vi "5492_WPI_RobotDriveArcadeDrive_Standard(NoSaturation).vi"(0 "RobotDriveDevRef":T1={"DevStatus"={"status"=FALSE, "code"=0, "source"=""}, "Motors[]"=[], "Square Inputs"=FALSE, "Max Output"=1.0}, 5 "X axis value":dbl, 7 "Orientation Toggle":bool, 9 "Y axis value":dbl, 11 "error in (no error)":errorcluster) -> (4 "RobotDriveDevRef":T1={"DevStatus"={"status"=FALSE, "code"=0, "source"=""}, "Motors[]"=[], "Square Inputs"=FALSE, "Max Output"=1.0}, 6 "Motor Values":dbl[](array[numeric]), 15 "error out":errorcluster)   [LabVIEW 2016]
doc: "Uses a standard algorithm to configure the motors for arcade driving. This algorithm does not saturate over half of the range.\n\nThis software is licensed. Open the labview\\readme\\WPI Robotics Library Open Source License.txt file for more information."
uses:
  <vilib>/Rock Robotics/WPI/RobotDrive/WPI_RobotDriveDevRef.ctl
  <vilib>/Rock Robotics/WPI/MotorControl/WPI_MotorControlDeviceRef.ctl
  <vilib>/Rock Robotics/WPI/MotorControl/WPI_MotorControlType.ctl
  <vilib>/Rock Robotics/SystemInterfaces/DIO/FPGA_DIOPWMChannel.ctl
  <vilib>/Rock Robotics/WPI/PWM/WPI_PWMDeadband.ctl
  <vilib>/Rock Robotics/SystemInterfaces/NetworkCommunication/NetComm_UsageReport_ResourceType.ctl
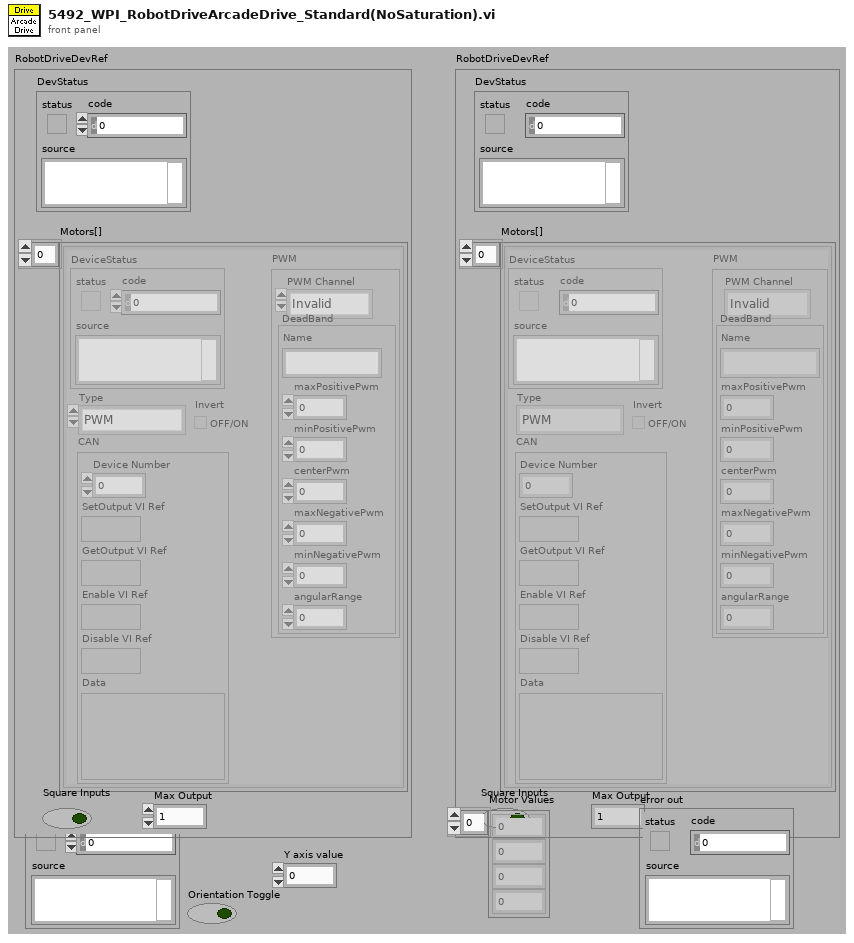
[diagram p1: front panel]
types:
  T1 = typedef "WPI_RobotDriveDevRef.ctl" = cluster{"DevStatus":errorcluster, "Motors[]":T2[], "Square Inputs":bool, "Max Output":dbl}
  T2 = typedef "WPI_MotorControlDeviceRef.ctl" = cluster{"DeviceStatus":errorcluster, "Type":T3, "PWM":cluster{"PWM Channel":T4, "DeadBand":T5}, "CAN":cluster{"Device Number":u8, "SetOutput VI Ref":variant, "GetOutput VI Ref":variant, "Enable VI Ref":variant, "Disable VI Ref":variant, "Data":variant}, "Invert":bool}
  T3 = typedef "WPI_MotorControlType.ctl" = enum16{"PWM", "CAN"}
  T4 = typedef "FPGA_DIOPWMChannel.ctl" = enum8{"PWM 0", "PWM 1", "PWM 2", "PWM 3", "PWM 4", "PWM 5", "PWM 6", "PWM 7", "PWM 8", "PWM 9", "PWM MXP 0", "PWM MXP 1", "PWM MXP 2", "PWM MXP 3", "PWM MXP 4", "PWM MXP 5", "PWM MXP 6", "PWM MXP 7", "PWM MXP 8", "PWM MXP 9", "Invalid"}
  T5 = typedef "WPI_PWMDeadband.ctl" = cluster{"Name":string, "maxPositivePwm":i32, "minPositivePwm":i32, "centerPwm":i32, "maxNegativePwm":i32, "minNegativePwm":i32, "angularRange":u16}
  T6 = typedef "NetComm_UsageReport_ResourceType.ctl" = enum8{"Controller", "Module", "Language", "CANPlugin", "Accelerometer", "ADXL345", "AnalogChannel", "AnalogTrigger", "AnalogTriggerOutput", "CANJaguar", "Compressor", "Counter", "Dashboard", "DigitalInput", "DigitalOutput", "DriverStationCIO", "DriverStationEIO", "DriverStationLCD", "Encoder", "GearTooth", "Gyro", "I2C", "Framework", "Jaguar", "Joystick", "Kinect", "KinectStick", "PIDController", "Preferences", "PWM", "Relay", "RobotDrive", "SerialPort", "Servo", "Solenoid", "SPI", "Task", "Ultrasonic", "Victor", "Button", "Command", "AxisCamera", "PCVideoServer", "SmartDashboard", "Talon", "HiTechnicColorSensor", "HiTechnicAccel", "HiTechnicCompass", "SRF08", "AnalogOutput", "Victor SP", "Talon SRX", "CAN Talon SRX", "ADXL362 Accel", "ADXRS450 Gyro", "Rev SPARK", "Mindsensors SD540", "Digital Filter", "ADIS16448", "PDP", "PCM", "PigeonIMU"}
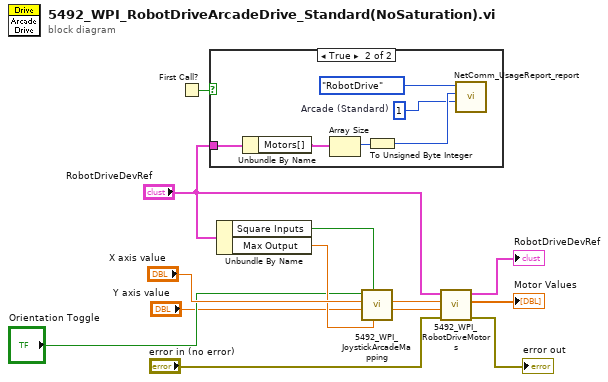
[diagram p0: block diagram]
diagram:
  n1 = First Call?() -> (First Call?: T/F=w10:bool)
  n2 = case shown="True" w10 {
    tunnel: "RobotDriveDevRef" -> [_ w15]
    frame False {
    }
    frame True {
      w17 = u8 1  # Arcade (Standard)
      n3 = Unbundle By Name(w15) -> ("Motors[]"=w14:T2[])
      n4 = Array Size(array=w14) -> (size(s)=w16:i32)
      n5 = To Unsigned Byte Integer(number=w16) -> (unsigned 8bit integer=w18:u8)
      n6 = call <vilib>:"NetComm_UsageReport_report.vi"("Context"=w17, "Instance Number"=w18, "Resource Type"=NetComm_UsageReport_ResourceType."RobotDrive") -> ()  [unwired: 9 in]
    }
  }
  n7 = Unbundle By Name("RobotDriveDevRef") -> ("Square Inputs"=w6:bool, "Max Output"=w4:dbl)
  n8 = call "5492_WPI_JoystickArcadeMapping.vi"("Max Output"=w4, "Square Inputs"=w6, "Y axis value"="Y axis value", "X axis value"="X axis value", "Orientation Toggle"="Orientation Toggle") -> ("Right Motor Value"=w7:dbl, "Left Motor Value"=w8:dbl)  [unwired: 5 in]
  n9 = call "5492_WPI_RobotDriveMotors.vi"("error in (no error)"="error in (no error)", "RightSpeed"=w7, "LeftSpeed"=w8, "RobotDriveDevRef"="RobotDriveDevRef") -> ("error out"=→"error out":errorcluster, "Motor Values"=→"Motor Values":dbl[], "RobotDriveDevRef"=→"RobotDriveDevRef":T1)  [unwired: 5 out]
